vi "CapacitanceSimple.vi"() -> ()   [LabVIEW 2015]
panel:
  out "Loss":dbl format="%.8f"
  out "Capacitance":dbl format="%.8f"
  out "Numeric":i32
  out "XY Graph":cluster{dbl[], dbl[]}(graph)
  out "File:":string
  out "Path":path
  out "error out":errorcluster
  in  "error in (no error)":errorcluster
  in  "Capacitance Bridge\nAddress:":i16=28
  in  "Magnet Power Supply\nAddress:":i16=24
  in  "stop":bool
  in  "Plot on Y-axis:":u16(ring) items=["Loss", "Capascitance", "Loss", "Field", "Capacitance"]
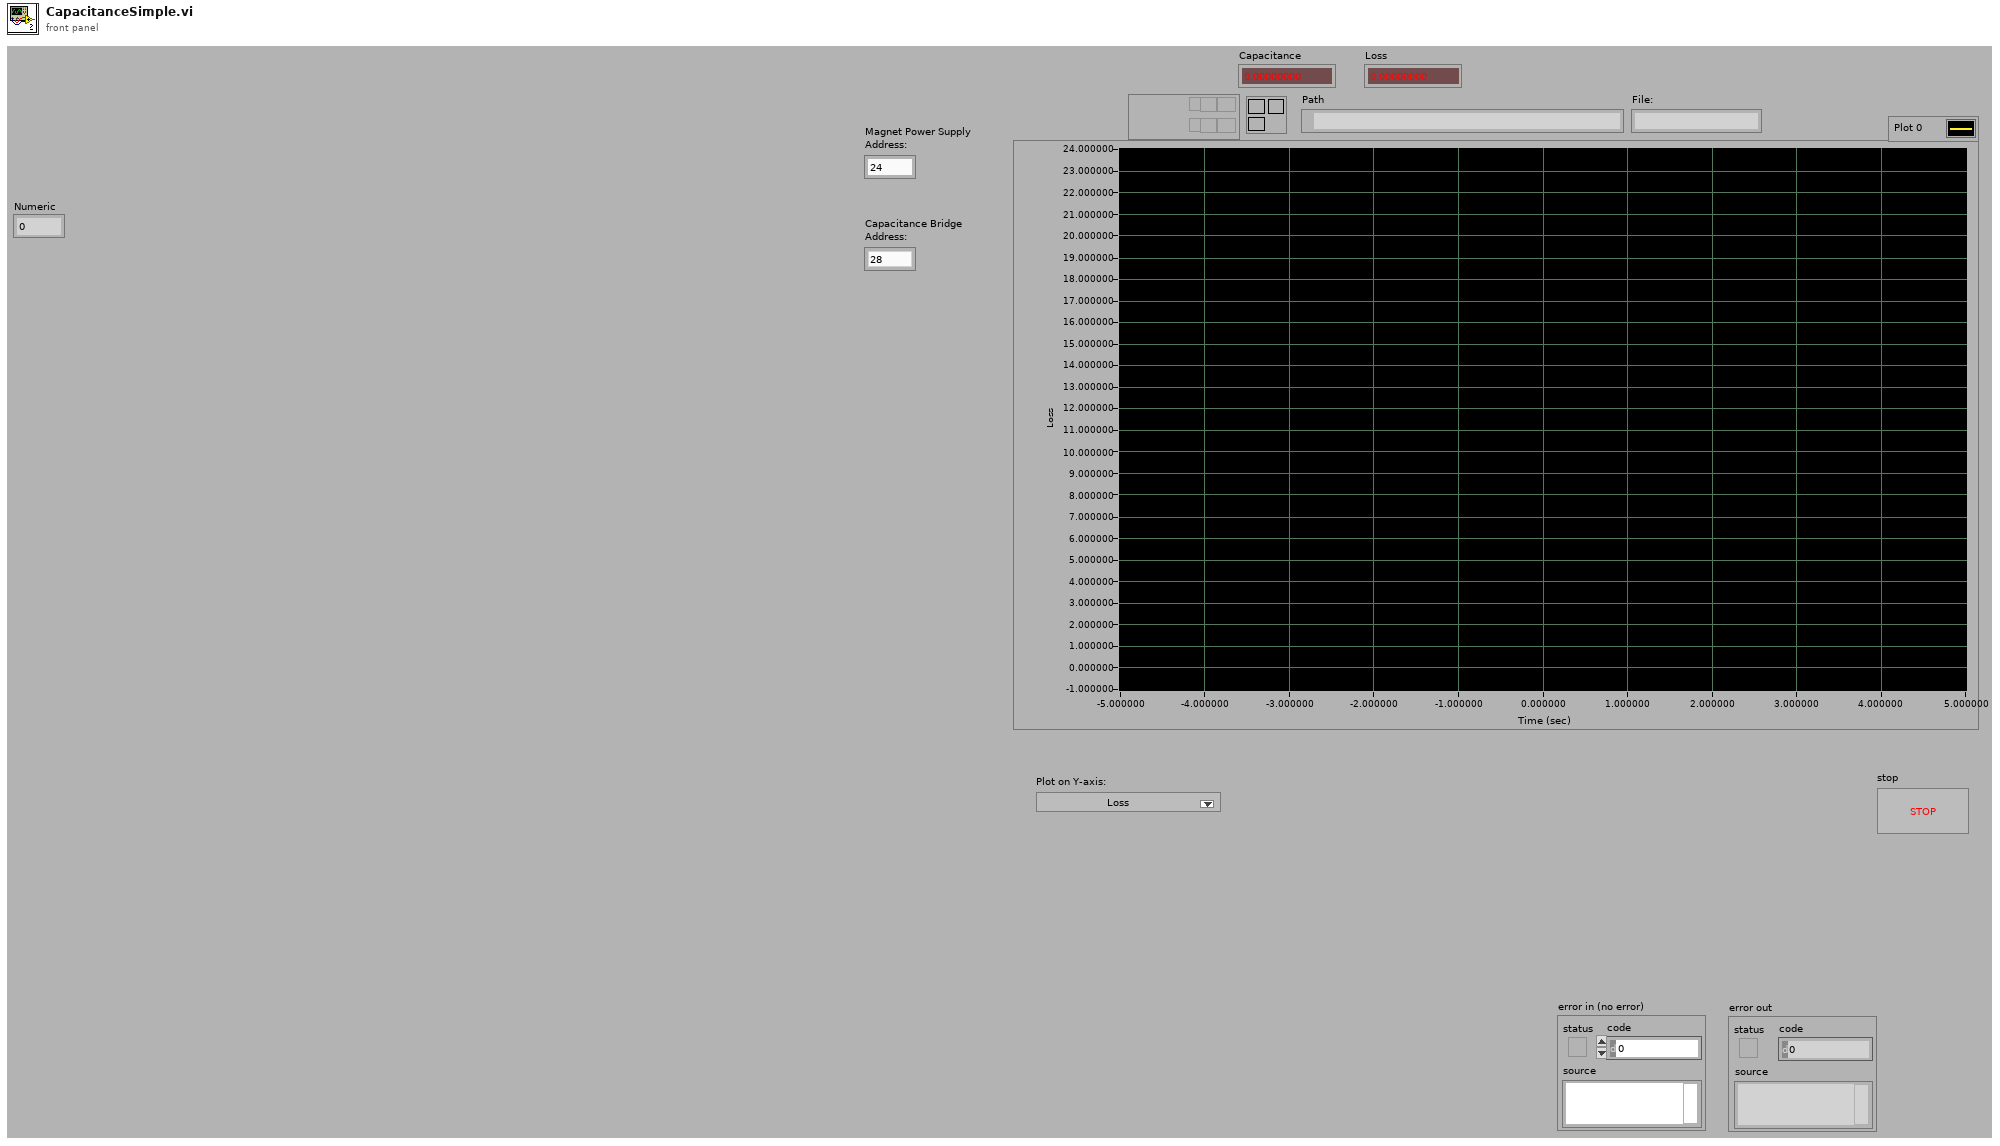
[diagram p1: front panel]
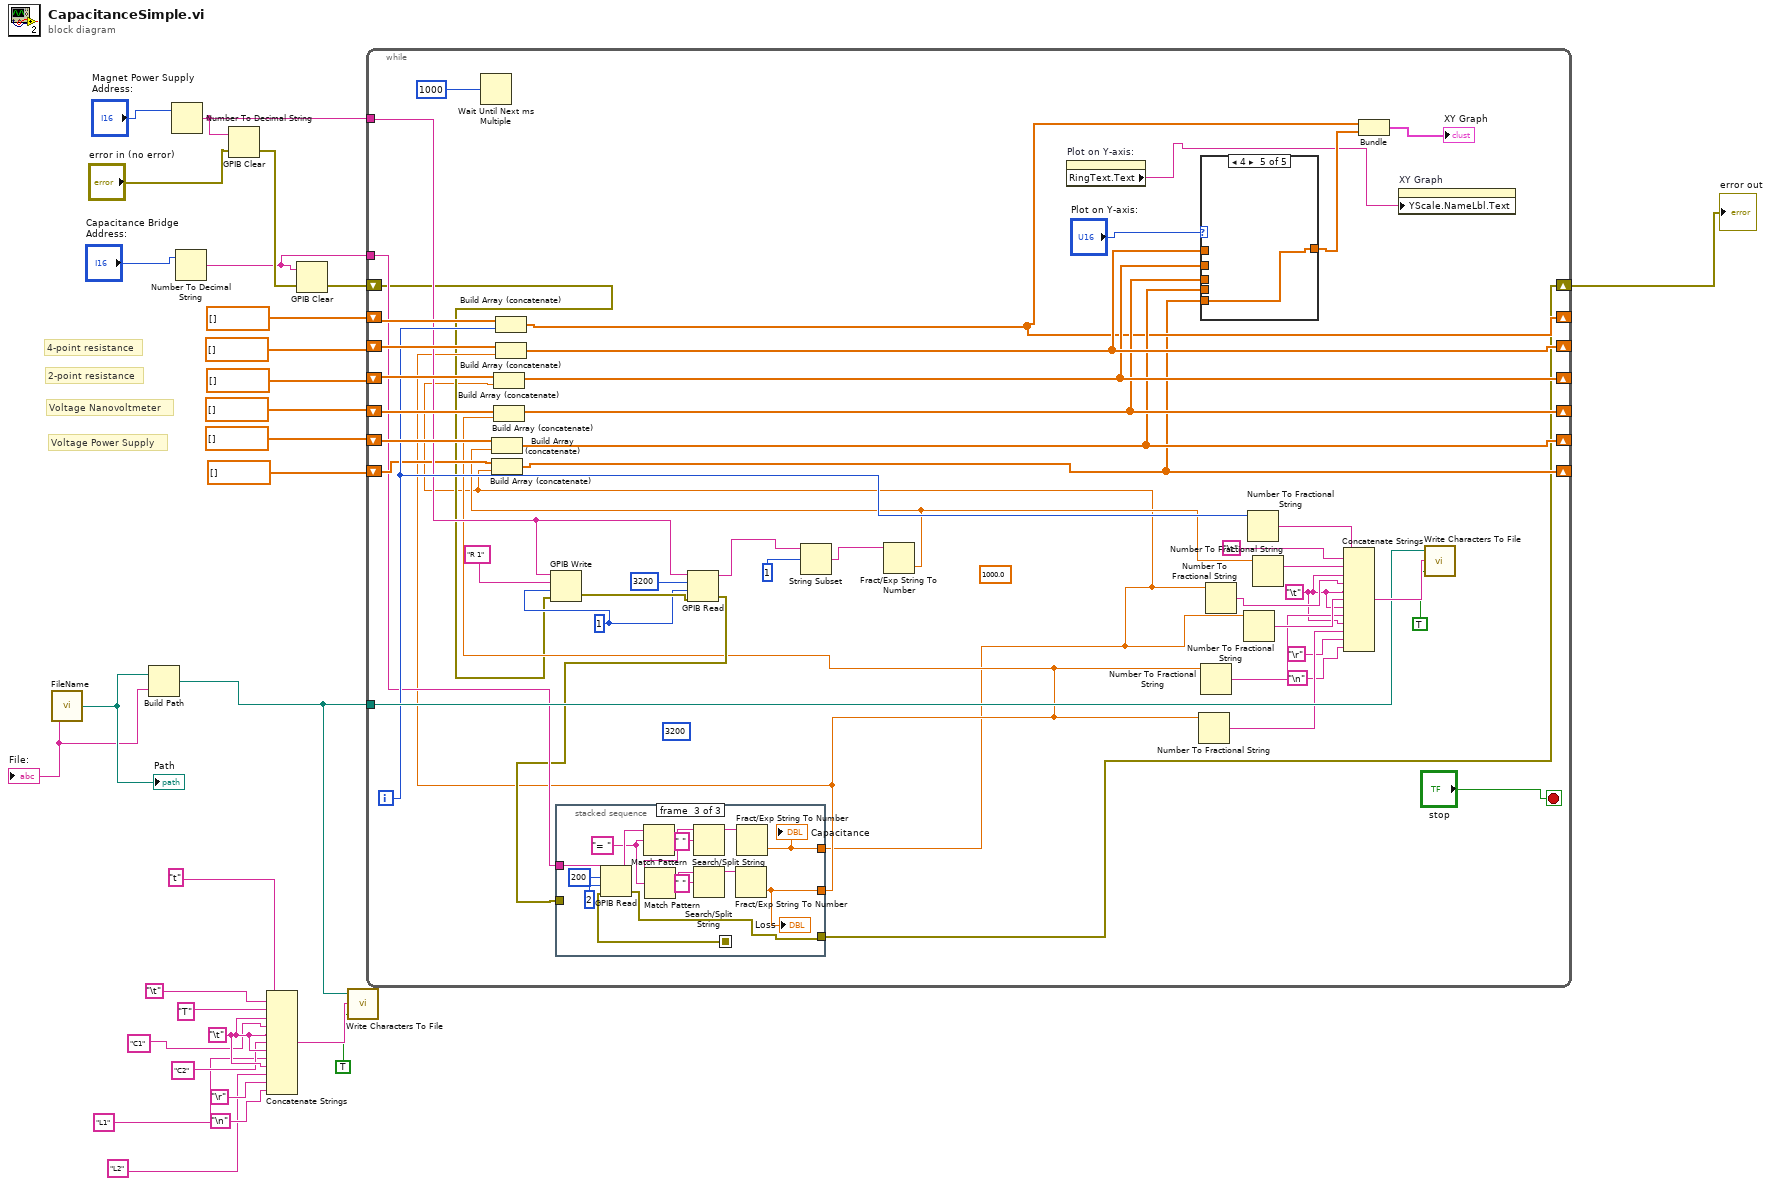
[diagram p0: block diagram]
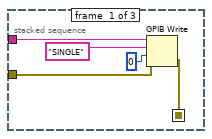
[diagram p2: hidden frame]
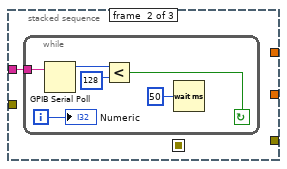
[diagram p3: hidden frame]
diagram:
  w11 = "\t"
  # "Voltage Power Supply"
  # "Voltage Nanovoltmeter"
  # "2-point resistance"
  # "4-point resistance"
  n1 = call "FileName.vi"() -> ("dup directory path"=w23:path, "String"=w22:string)
  "Path" <- w23
  "File:" <- w22
  n2 = Build Path(base path=w23, name or relative path=w22) -> (appended path=w7:path)
  n3 = Number To Decimal String(number="Magnet Power Supply\nAddress:") -> (decimal integer string=w25:string)  [unwired: 1 in]
  n4 = Number To Decimal String(number="Capacitance Bridge\nAddress:") -> (decimal integer string=w15:string)  [unwired: 1 in]
  n5 = GPIB Clear(2:"error in (no error)", 3:w25) -> (0:w27:errorcluster)  [unwired: 1 out]
  n6 = Concatenate Strings("t", "\t", "T", w11, "C1", w11, "C2", w11, "L1", w11, "L2", "\r", "\n") -> (w13:string)
  n7 = GPIB Clear(2:w27, 3:w15) -> (0:w24:errorcluster)  [unwired: 1 out]
  n8 = call <vilib>:"Write Characters To File.vi"("append to file? (new file:F)"=TRUE, "character string"=w13, "file path (dialog if empty)"=w7) -> ()  [unwired: 2 in, 1 out]
  n9 = while {
    tunnel: w25 -> [w43]
    tunnel: w7 -> [w67]
    shift-right: [w50] -> _
    shift-left: dbl[] [] -> [w55]
    shift-right: [w49] -> _
    shift-left: dbl[] [] -> [w56]
    shift-right: [w48] -> _
    shift-left: dbl[] [] -> [w64]
    shift-right: [w47] -> _
    shift-left: dbl[] [] -> [w65]
    shift-right: [w38] -> w17
    shift-left: w24 -> [w35]
    shift-right: [w45] -> _
    shift-left: dbl[] [] -> [w53]
    tunnel: w15 -> [w40]
    shift-right: [w41] -> _
    shift-left: dbl[] [] -> [w42]
    i -> [w52]
    stop <- "stop" stop-if-true
    w36 = 1
    (unwired) 1000.0
    w59 = "\t"
    (unwired) 3200
    n10 = Wait Until Next ms Multiple(millisecond multiple=1000) -> ()  [unwired: 1 out]
    n11 = Build Array (concatenate)(w53, w52) -> (w45:dbl[])
    n12 = GPIB Write(0:w43, 1:"R 1", 2:w36, 3:w35) -> (6:w75:errorcluster)  [unwired: 1 in, 1 out]
    n13 = GPIB Read(0:w43, 1:3200, 2:w36, 3:w75) -> (5:w33:string, 7:w39:errorcluster)  [unwired: 1 in, 1 out]
    n14 = stacked-sequence {
      seq-local: [w77 _ _] -> [_ _ w100]
      tunnel: w40 -> [w80 w82 w101]
      tunnel: w39 -> [w78 _ _]
      tunnel: [_ _ w94] -> w37
      tunnel: [_ _ w95] -> w30
      tunnel: [_ _ w89] -> w38
      frame #0 {
        n15 = GPIB Write(0:w80, 1:"SINGLE" ("data"), 2:i16 0 ("mode (0)"), 3:w78) -> (6:w77:errorcluster)  [unwired: 1 in, 1 out]
      }
      frame #1 {
        n16 = while {
          tunnel: w82 -> [w88]
          i -> [w83]
          stop <- w85 continue-if-true
          n17 = GPIB Serial Poll(0:w88) -> (2:w87:i16)  [unwired: 1 in, 2 out]
          n18 = Less?(x=w87, y=i16 128) -> (x < y?=w85:bool)
          n19 = Wait (ms)(milliseconds to wait=u32 50) -> ()  [unwired: 1 out]
          "Numeric" <- w83
        }
      }
      frame #2 {
        w91 = "= "
        n20 = GPIB Read(0:w101, 1:200 ("byte count"), 2:i16 2 ("mode (0)"), 3:w100) -> (5:w93:string, 7:w89:errorcluster)  [unwired: 1 in, 1 out]
        n21 = Match Pattern(string=w93, regular expression=w91) -> (after substring=w92:string)  [unwired: 1 in, 3 out]
        n22 = Match Pattern(string=w92, regular expression=w91) -> (after substring=w90:string)  [unwired: 1 in, 3 out]
        n23 = Search/Split String(string=w92, search string/char (-)=" ") -> (substring before match=w97:string)  [unwired: 1 in, 2 out]
        n24 = Search/Split String(string=w90, search string/char (-)=" ") -> (substring before match=w96:string)  [unwired: 1 in, 2 out]
        n25 = Fract/Exp String To Number(string=w96) -> (number=w94:dbl)  [unwired: 3 in, 1 out]
        "Loss" <- w94
        n26 = Fract/Exp String To Number(string=w97) -> (number=w95:dbl)  [unwired: 3 in, 1 out]
        "Capacitance" <- w95
      }
    }
    n27 = Build Array (concatenate)(w42, w30) -> (w41:dbl[])
    n28 = Build Array (concatenate)(w56, w30) -> (w49:dbl[])
    n29 = Build Array (concatenate)(w64, w37) -> (w48:dbl[])
    n30 = Build Array (concatenate)(w55, w37) -> (w50:dbl[])
    n31 = String Subset(string=w33, offset (0)=1) -> (substring=w32:string)  [unwired: 1 in]
    n32 = Fract/Exp String To Number(string=w32) -> (number=w31:dbl)  [unwired: 3 in, 1 out]
    n33 = Build Array (concatenate)(w65, w31) -> (w47:dbl[])
    n34 = property on="Plot on Y-axis:" class="Ring (strict)"() -> ("RingText.Text"=w44:string)  [unwired: 2 in, 2 out]
    n35 = Number To Fractional String(number=w37) -> (F-format string=w60:string)  [unwired: 3 in]
    n36 = case shown="4" "Plot on Y-axis:" {
      tunnel: w50 -> [w104 _ _ _ _]
      tunnel: w49 -> [_ w105 _ _ _]
      tunnel: w48 -> [_ _ w106 _ _]
      tunnel: w47 -> [_ _ _ w107 _]
      tunnel: [w104 w105 w106 w107 w108] -> w46
      tunnel: w41 -> [_ _ _ _ w108]
      frame 0, Default {
      }
      frame 1 {
      }
      frame 2 {
      }
      frame 3 {
      }
      frame 4 {
      }
    }
    n37 = Number To Fractional String(number=w37) -> (F-format string=w61:string)  [unwired: 3 in]
    n38 = Number To Fractional String(number=w30) -> (F-format string=w63:string)  [unwired: 3 in]
    n39 = Number To Fractional String(number=w30) -> (F-format string=w62:string)  [unwired: 3 in]
    n40 = Number To Fractional String(number=w52) -> (F-format string=w72:string)  [unwired: 3 in]
    n41 = Number To Fractional String(number=w31) -> (F-format string=w68:string)  [unwired: 3 in]
    n42 = Concatenate Strings(w72, "\t", w68, w59, w63, w59, w62, w59, w61, w59, w60, "\r", "\n") -> (w70:string)
    n43 = Bundle(w45, w46) -> (→"XY Graph":cluster{dbl[], dbl[]})  [unwired: 1 in]
    n44 = property on="XY Graph" class="XYGraph (strict)"("YScale.NameLbl.Text"=w44) -> ()  [unwired: 2 in, 2 out]
    n45 = call <vilib>:"Write Characters To File.vi"("append to file? (new file:F)"=TRUE, "character string"=w70, "file path (dialog if empty)"=w67) -> ()  [unwired: 2 in, 1 out]
  }
  "error out" <- w17
